vi "camera_settings.vi"() -> (3 "Camera settings output":T1={"Gain"=1.0, "Exposure (s)"=0.05, "Preview binning"=2, "Capture binning"=0} {"Capture binning" items=["1x1", "2x2", "4x4", "8x8"]; "Preview binning" items=["1x1", "2x2", "4x4", "8x8"]; "Exposure (s)" scale=1e-05..1000.0 scale format="%^#_1e"; "Gain" scale=0.451..21.5 scale format="%#_3g"})   [LabVIEW 2011]
uses:
  typedefs/camera_settings.ctl
  <vilib>/vision/NI_Vision_Development_Module.lvlib
panel:
  in  "auto expose button":bool
  out "Histogram":T2(graph)
  in  "Camera settings":T1={"Gain"=1.0, "Exposure (s)"=0.05, "Preview binning"=2, "Capture binning"=0} {"Capture binning" items=["1x1", "2x2", "4x4", "8x8"]; "Preview binning" items=["1x1", "2x2", "4x4", "8x8"]; "Exposure (s)" scale=1e-05..1000.0 scale format="%^#_1e"; "Gain" scale=0.451..21.5 scale format="%#_3g"}
  out "error out":errorcluster
  in  "close preview button":bool
  out "Preview":T3(plugin-control)
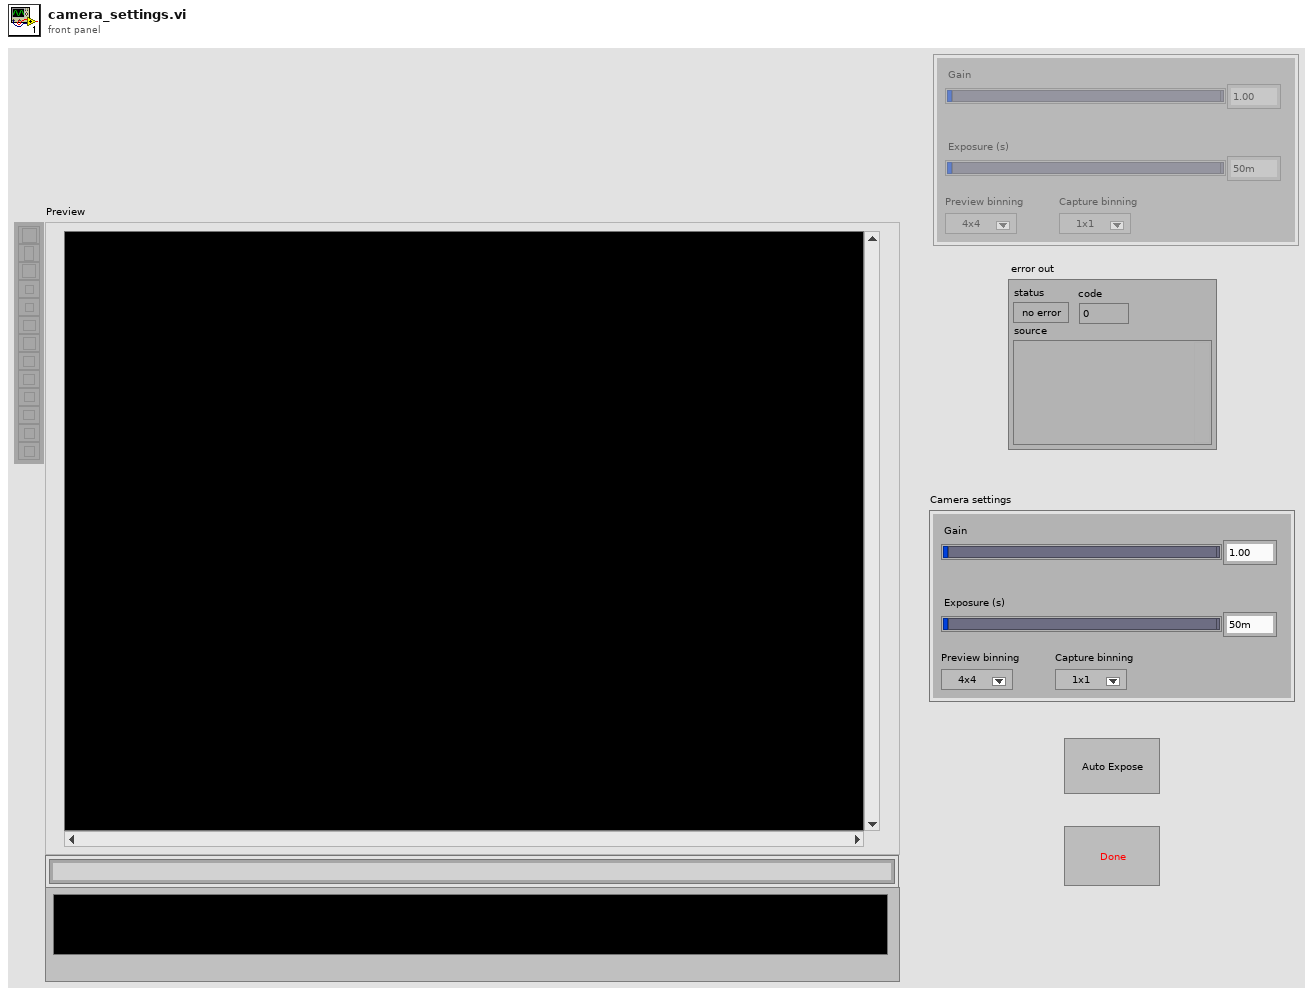
[diagram p1: front panel]
types:
  T1 = typedef "camera_settings.ctl" = cluster{"Gain":dbl, "Exposure (s)":dbl, "Preview binning":u16, "Capture binning":u16}
  T2 = cluster{"Starting Value":sgl, "Incremental Value":sgl, "Histogram":u32[]}
  T3 = typedef "IMAQ Image.ctl" = refnum<image>
  T4 = typedef "Image Type" = u32
  T5 = enum32{"gain", "offset", "exposure", "binning", "horizontal binning", "vertical binning", "readout speed", "trigger type", "lcd filter", "cooler", "exposure red", "exposure blue", "image format", "roi x", "roi y", "roi width", "roi height", "reserved1", "shutter state", "reserved2", "sync-b out", "reserved3", "intensifier gain", "trigger delay", "camera mode", "normalized gain", "normalized intenifier gain DB", "doPostProcessing", "postProcessGainRed", "postProcessGainGreen", "postProcessGainBlue", "postProcessBayerAlgorithm", "postProcessImageFormat", "fan", "blackout mode", "high sensitivity", "Readout Port", "EM Gain", "open delay", "close delay", "clearing mode"}
  T6 = cluster{"Global Rectangle":i32[], "Contours":cluster{"Contour Type":u32, "ROI Type":u32, "Points":i32[]}[]}
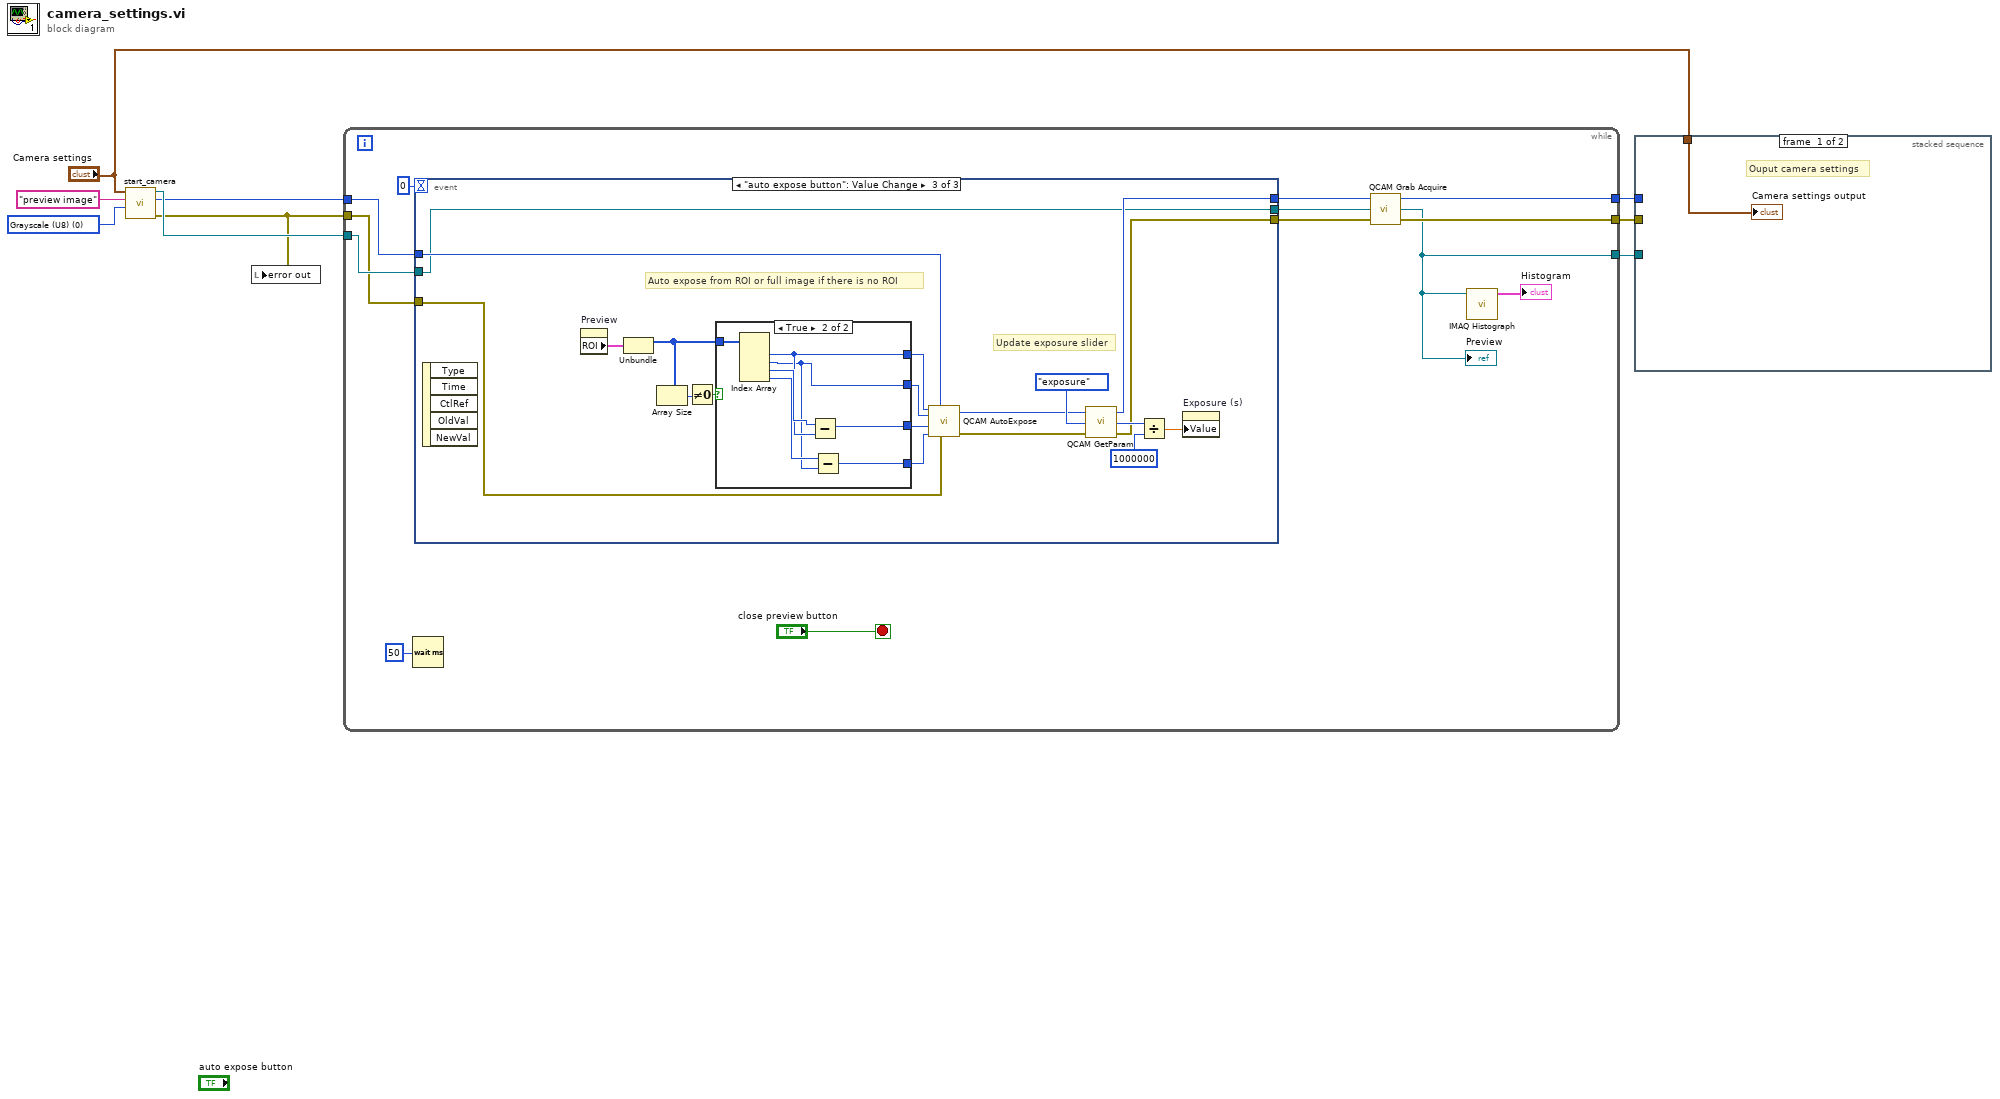
[diagram p0: block diagram]
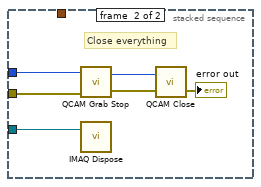
[diagram p2: hidden frame]
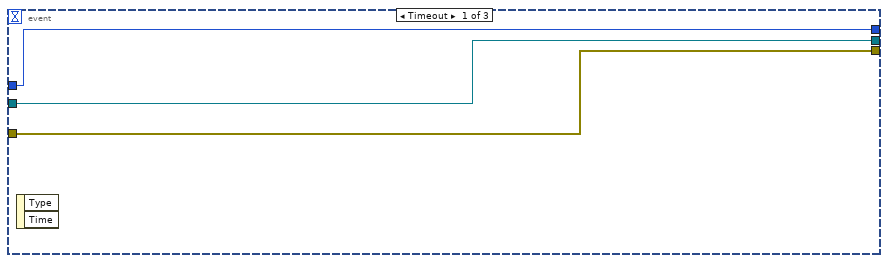
[diagram p3: hidden frame]
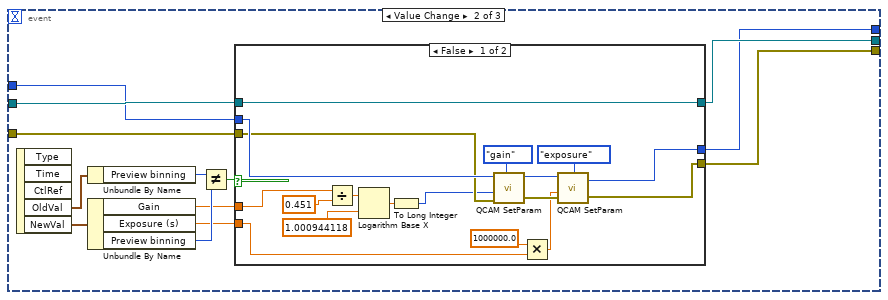
[diagram p4: hidden frame]
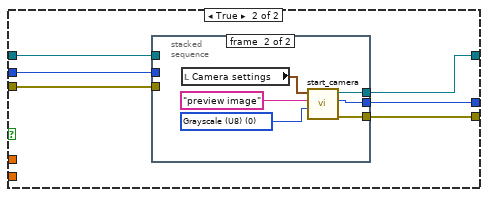
[diagram p5: hidden frame]
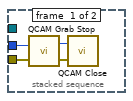
[diagram p6: hidden frame]
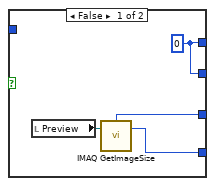
[diagram p7: hidden frame]
diagram:
  w6 = T4 0 items=["Grayscale (U8)", "Grayscale (I16)", "Grayscale (SGL)", "Complex (CSG)", "RGB (U32)", "HSL (U32)", "RGB (U64)"] ("Image Type")
  n1 = call "start_camera.vi"("Image Type"=w6, "String"="preview image", "Camera settings"="Camera settings") -> ("error out"=w2:errorcluster, "cameraId out"=w3:u32, "Refnum out"=w4:T3)  [unwired: 6 in]
  n2 = local write "error out"(w2) -> ()
  n3 = while {
    tunnel: w3 -> [w14]
    tunnel: w2 -> [w15]
    tunnel: w4 -> [w16]
    tunnel: [w22] -> w9
    tunnel: [w21] -> w8
    tunnel: [w17] -> w7
    stop <- "close preview button" stop-if-true
    n4 = Wait (ms)(milliseconds to wait=u32 50) -> ()  [unwired: 1 out]
    n5 = event shown="[2] \"auto expose button\": Value Change" {
      selector: _ -> [_ _ _]
      dyn-events: _ -> [_ _ _]
      timeout: 0 -> [_ _ _]
      tunnel: w16 -> [w24 w33 w76]
      tunnel: w15 -> [w23 w30 w73]
      tunnel: w14 -> [w25 w29 w79]
      tunnel: [w25 w27 w77] -> w13
      tunnel: [w24 w28 w76] -> w12
      tunnel: [w23 w26 w75] -> w11
      event Timeout {
        n6 = event-data() -> ()  [unwired: 1 in, 2 out]
      }
      event Value Change {
        n7 = event-data() -> ("OldVal"=w37:T1, "NewVal"=w38:T1)  [unwired: 1 in, 3 out]
        n8 = Unbundle By Name(w37) -> ("Preview binning"=w36:u16)
        n9 = Unbundle By Name(w38) -> ("Gain"=w32:dbl, "Exposure (s)"=w31:dbl, "Preview binning"=w34:u16)
        n10 = Not Equal?(x=w34, y=w36) -> (x != y?=w35:bool)
        n11 = case shown="False" w35 {
          tunnel: w30 -> [w45 w62]
          tunnel: w33 -> [w56 w61]
          tunnel: [w56 w60] -> w28
          tunnel: w32 -> [w39 _]
          tunnel: w31 -> [w49 _]
          tunnel: w29 -> [w48 w59]
          tunnel: [w47 w58] -> w27
          tunnel: [w46 w57] -> w26
          frame False {
            n12 = Divide(x=w39, y=0.451) -> (x/y=w43:dbl)
            n13 = Logarithm Base X(1:1.000944118 ("x"), 2:w43) -> (0:w41:dbl)
            n14 = To Long Integer(number=w41) -> (32bit integer=w40:i32)
            n15 = call <userlib>:"QCAM SetParam.vi"("error in (no error)"=w45, "value"=w40, "parameter key"=T5."gain", "cameraId"=w48) -> ("error out"=w54:errorcluster, "cameraId out"=w53:u32)
            n16 = Multiply(x=1000000.0, y=w49) -> (x*y=w52:dbl)
            n17 = call <userlib>:"QCAM SetParam.vi"("error in (no error)"=w54, "value"=w52, "parameter key"=T5."exposure", "cameraId"=w53) -> ("error out"=w46:errorcluster, "cameraId out"=w47:u32)
          }
          frame True {
            n18 = stacked-sequence {
              tunnel: w62 -> [w64 _]
              tunnel: w61 -> [_ _]
              tunnel: [_ w69] -> w60
              tunnel: w59 -> [w63 _]
              tunnel: [_ w68] -> w58
              tunnel: [_ w67] -> w57
              frame #0 {
                n19 = call <userlib>:"QCAM Grab Stop.vi"("error in (no error)"=w64, "cameraId"=w63) -> ("error out"=w65:errorcluster, "cameraId Out"=w66:u32)
                n20 = call <userlib>:"QCAM Close.vi"("error in (no error)"=w65, "cameraId"=w66) -> ()  [unwired: 1 in, 1 out]
              }
              frame #1 {
                w72 = T4 0 items=["Grayscale (U8)", "Grayscale (I16)", "Grayscale (SGL)", "Complex (CSG)", "RGB (U32)", "HSL (U32)", "RGB (U64)"] ("Image Type")
                n21 = local read "Camera settings"() -> (w70:T1)
                n22 = call "start_camera.vi"("Image Type"=w72, "String"="preview image", "Camera settings"=w70) -> ("error out"=w67:errorcluster, "cameraId out"=w68:u32, "Refnum out"=w69:T3)  [unwired: 6 in]
              }
            }
          }
        }
      }
      event "auto expose button": Value Change {
        # "Auto expose from ROI or full image if there is no ROI"
        # "Update exposure slider"
        n23 = event-data() -> ()  [unwired: 1 in, 5 out]
        n24 = property on="Preview" class="ImageControl"() -> ("ROI"=w80:T6)  [unwired: 2 in, 2 out]
        n25 = Unbundle(w80) -> ("Global Rectangle"=w81:i32[])  [unwired: 1 out]
        n26 = Array Size(array=w81) -> (size(s)=w82:i32)
        n27 = Not Equal To 0?(x=w82) -> (x != 0?=w83:bool)
        n28 = case shown="True" w83 {
          tunnel: w81 -> [_ w100]
          tunnel: [w92 w99] -> w84
          tunnel: [w92 w98] -> w85
          tunnel: [w93 w97] -> w86
          tunnel: [w94 w96] -> w87
          frame False {
            w92 = 0
            n29 = local read "Preview"() -> (w95:T3)
            n30 = call "IMAQ GetImageSize"("Image"=w95) -> ("Y Resolution"=w94:i32, "X Resolution"=w93:i32)  [unwired: 3 in, 1 out]
          }
          frame True {
            n31 = Index Array(array=w100) -> (element #1=w99:i32, element #2=w98:i32, element #3=w102:i32, element #4=w101:i32)  [unwired: 4 in]
            n32 = Subtract(x=w102, y=w99) -> (x-y=w97:i32)
            n33 = Subtract(x=w101, y=w98) -> (x-y=w96:i32)
          }
        }
        n34 = call <userlib>:"QCAM AutoExpose.vi"("xOrig"=w84, "cameraId"=w79, "yOrig"=w85, "width"=w86, "error in (no error)"=w73, "height"=w87) -> ("cameraId out"=w78:u32, "error out"=w74:errorcluster)  [unwired: 1 in]
        n35 = call <userlib>:"QCAM GetParam.vi"("cameraId in"=w78, "parameter key"=T5."exposure", "error in (no error)"=w74) -> ("cameraId out"=w77:u32, "value out"=w88:u32, "error out"=w75:errorcluster)  [unwired: 2 out]
        n36 = Divide(x=w88, y=1000000) -> (x/y=w91:dbl)
        n37 = property on="Exposure (s)" class="Slide (strict)"("Value"=w91) -> ()  [unwired: 2 in, 2 out]
      }
    }
    n38 = call <userlib>:"QCAM Grab Acquire.vi"("error in (no error)"=w11, "Image"=w12, "cameraId"=w13) -> ("error out"=w21:errorcluster, "Image Out"=w17:T3, "cameraId out"=w22:u32)
    "Preview" <- w17
    n39 = call "IMAQ Histograph"("Image"=w17) -> ("Histogram Graph"=→"Histogram":T2)  [unwired: 7 in, 3 out]
  }
  n40 = stacked-sequence {
    tunnel: w9 -> [_ w109]
    tunnel: w8 -> [_ w108]
    tunnel: w7 -> [_ w107]
    tunnel: "Camera settings" -> [w103 _]
    frame #0 {
      # "Ouput camera settings"
      "Camera settings output" <- w103
    }
    frame #1 {
      # "Close everything"
      n41 = call <userlib>:"QCAM Grab Stop.vi"("error in (no error)"=w108, "cameraId"=w109) -> ("error out"=w105:errorcluster, "cameraId Out"=w106:u32)
      n42 = call "IMAQ Dispose"("Image"=w107) -> ()  [unwired: 5 in, 1 out]
      n43 = call <userlib>:"QCAM Close.vi"("error in (no error)"=w105, "cameraId"=w106) -> ("error out"=→"error out":errorcluster)  [unwired: 1 in]
    }
  }
